vi "Has Next.vi"(8 "error in (no error)":errorcluster, 11 "Scanner.lvclass in":refnum<class "Scanner.lvclass">) -> (0 "error out":errorcluster, 2 "Again?":bool, 3 "Scanner.lvclass out":refnum<class "Scanner.lvclass">)   [LabVIEW 2012, in "Scanner.lvclass"]
doc: "(Dynamic) Return TRUE if this Scanner has not yet completed all steps in its preconfigured Range."
uses:
  Scanner.lvclass
  Scanner.lvclass/Scanner.ctl
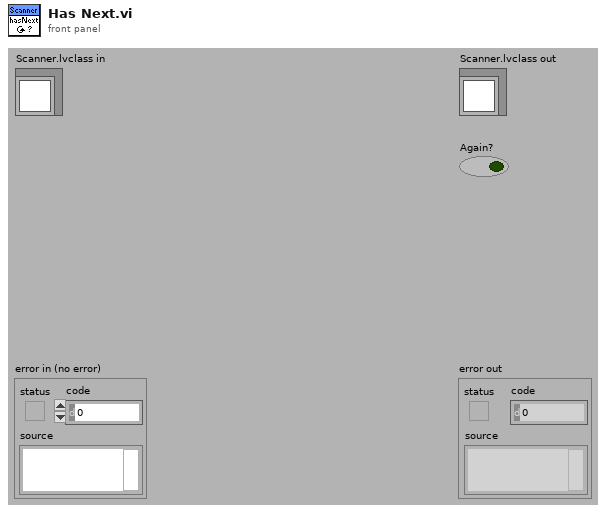
[diagram p1: front panel]
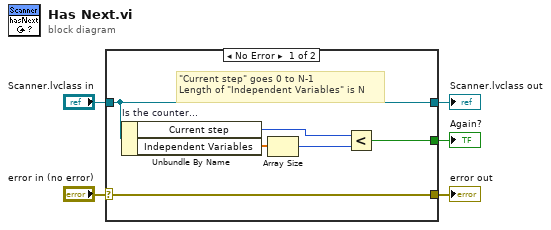
[diagram p0: block diagram]
diagram:
  n1 = case shown="No Error" "error in (no error)" {
    selector: "error in (no error)" -> [w11 w12]
    tunnel: [w11 w12] -> w4
    tunnel: [w10 w13] -> w2
    tunnel: "Scanner.lvclass in" -> [w10 w13]
    tunnel: [w9 _] -> w1
    frame No Error {
      # "\"Current step\" goes 0 to N-1\nLength of \"Independent Variables\" is N"
      n2 = Unbundle By Name "Is the counter..."(w10) -> ("Current step"=w7:u32, "Independent Variables"=w8:dbl[])
      n3 = Array Size(array=w8) -> (size(s)=w6:i32)
      n4 = Less?(x=w7, y=w6) -> (x < y?=w9:bool)
    }
    frame Error {
    }
  }
  "error out" <- w4
  "Scanner.lvclass out" <- w2
  "Again?" <- w1
